vi "OrientationCW2(L).vi"() -> (0 "Array of Operations (out)":T1[](array[typedef])=[{"Device"=enum."Servo", "Angles"=[enum."0°", enum."-90°", enum."0°"], "Grips"=[]}, {"Device"=enum."Grip", "Angles"=[], "Grips"=[TRUE, FALSE, TRUE]}, {"Device"=enum."Servo", "Angles"=[enum."0°", enum."0°", enum."0°"], "Grips"=[]}, {"Device"=enum."Grip", "Angles"=[], "Grips"=[FALSE, TRUE, TRUE]}, {"Device"=enum."Servo", "Angles"=[enum."-90°", enum."0°", enum."0°"], "Grips"=[]}, {"Device"=enum."Grip", "Angles"=[], "Grips"=[TRUE, TRUE, FALSE]}, {"Device"=enum."Servo", "Angles"=[enum."-90°", enum."0°", enum."+90°"], "Grips"=[]}, {"Device"=enum."Grip", "Angles"=[], "Grips"=[TRUE, FALSE, TRUE]}, {"Device"=enum."Servo", "Angles"=[enum."0°", enum."0°", enum."0°"], "Grips"=[]}, {"Device"=enum."Grip", "Angles"=[enum."0°", enum."-90°", enum."0°"], "Grips"=[FALSE, TRUE, TRUE]}, {"Device"=enum."Servo", "Angles"=[enum."-90°", enum."0°", enum."0°"], "Grips"=[FALSE, FALSE, TRUE]}, {"Device"=enum."Grip", "Angles"=[enum."0°", enum."-90°", enum."0°"], "Grips"=[TRUE, TRUE]}, {"Device"=enum."Servo", "Angles"=[enum."-90°", enum."0°", enum."+90°"], "Grips"=[]}, {"Device"=enum."Grip", "Angles"=[enum."0°", enum."-90°", enum."0°"], "Grips"=[TRUE, FALSE, TRUE]}, {"Device"=enum."Servo", "Angles"=[enum."0°", enum."0°", enum."0°"], "Grips"=[]}, {"Device"=enum."Servo", "Angles"=[enum."0°", enum."-90°", enum."0°"], "Grips"=[]}, {"Device"=enum."Grip", "Angles"=[enum."0°", enum."-90°", enum."0°"], "Grips"=[TRUE, TRUE, TRUE]}])   [LabVIEW 2017]
uses:
  Projekt-RubikLibrary/RubikOps.ctl
  Projekt-RubikLibrary/ServoAbsAngleControl.ctl
  Projekt-RubikLibrary/RubikLibrary.lvlib
panel:
  in  "Array of Operations:  clockwise (cw) by 180°":T1[](array[typedef])=[{"Device"=enum."Grip", "Angles"=[], "Grips"=[FALSE, TRUE, TRUE]}, {"Device"=enum."Servo", "Angles"=[enum."-90°", enum."0°", enum."0°"], "Grips"=[]}, {"Device"=enum."Grip", "Angles"=[], "Grips"=[TRUE, TRUE, FALSE]}, {"Device"=enum."Servo", "Angles"=[enum."-90°", enum."0°", enum."+90°"], "Grips"=[]}, {"Device"=enum."Grip", "Angles"=[], "Grips"=[TRUE, FALSE, TRUE]}, {"Device"=enum."SyncTurn", "Angles"=[enum."0°", enum."0°", enum."0°"], "Grips"=[]}, {"Device"=enum."Grip", "Angles"=[], "Grips"=[FALSE, TRUE, TRUE]}, {"Device"=enum."Servo", "Angles"=[enum."-90°", enum."0°", enum."0°"], "Grips"=[]}, {"Device"=enum."Grip", "Angles"=[enum."0°", enum."-90°", enum."0°"], "Grips"=[TRUE, TRUE, FALSE]}, {"Device"=enum."Servo", "Angles"=[enum."-90°", enum."0°", enum."+90°"], "Grips"=[]}, {"Device"=enum."Grip", "Angles"=[enum."0°", enum."0°", enum."0°"], "Grips"=[TRUE, FALSE, TRUE]}, {"Device"=enum."SyncTurn", "Angles"=[enum."0°", enum."0°", enum."0°"], "Grips"=[]}, {"Device"=enum."Grip", "Angles"=[enum."0°", enum."0°", enum."0°"], "Grips"=[TRUE, TRUE, TRUE]}]
  # "Rotate Rubik's Cube"
  # "OrientationCW2(L).vi"
  # "Turn Cube clockwise twice (view from left servo or\ngreen face).\nUse in Orientation FSM.\nCompare to OrientationCCW2(L).vi"
  # "Remember:\n Right mouse click@Array > Data Operations \n> Make current value default\nbefore you can save your changes!"
  # "This is the first turn of the cube"
  # "This is the second  turn of the cube"
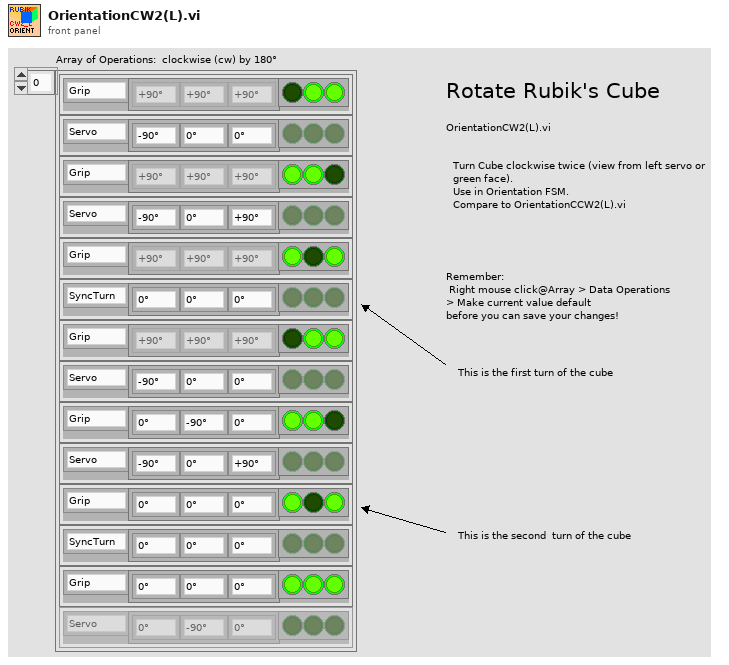
[diagram p1: front panel]
types:
  T1 = typedef "RubikLibrary.lvlib/RubikOps.ctl" = cluster{"Device":enum16{"Servo", "SyncTurn", "Grip"}, "Angles":T2[], "Grips":bool[]}
  T2 = typedef "RubikLibrary.lvlib/ServoAbsAngleControl.ctl" = enum16{"+90°", "0°", "-90°"}
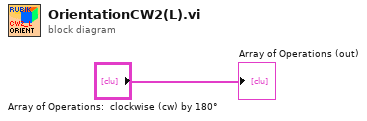
[diagram p0: block diagram]
diagram:
  "Array of Operations (out)" <- "Array of Operations:  clockwise (cw) by 180°"
